vi "Umgebung.ReadZustandsgrössen.vi"(0 "Umgebung in":refnum<data-value>, 5 "error in":errorcluster) -> (14 "Umgebung out":refnum<data-value>, 15 "Sekunden":dbl, 16 "Strahlungsleistung [W]":dbl, 17 "Solare Gewinne [W]":dbl, 18 "Aussentemperatur [°C]":dbl, 19 "error out":errorcluster)   [LabVIEW 2016, in "Umgebung.lvclass"]
uses:
  Umgebung.lvclass
  Umgebung.lvclass/Umgebung.ctl
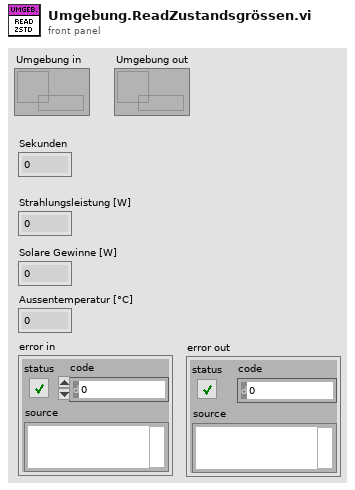
[diagram p1: front panel]
types:
  T1 = typedef "Umgebung.lvclass/Umgebung.Zustandsgrössen.ctl" = cluster{"Aussentemperatur [°C]":dbl, "Aussentemperatur [°C] Manuell":dbl, "Tag":dbl, "Stunde":dbl, "Minute":dbl, "Sekunden":dbl, "Strahlungsleistung [W/m2]":dbl, "Solare Gewinne [W/m2]":dbl, "Solare Gewinne [W/m2] Manuell":dbl, "Manuelle Eingabe On/Off":bool}
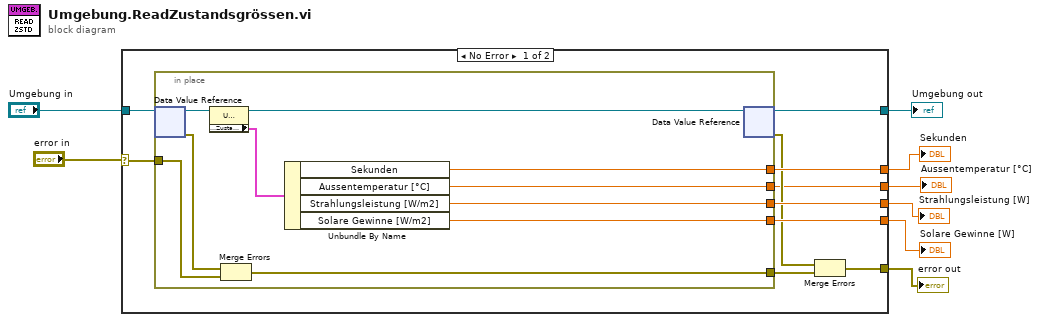
[diagram p0: block diagram]
diagram:
  n1 = case shown="No Error" "error in" {
    selector: "error in" -> [w11 w30]
    tunnel: [w18 _] -> w8
    tunnel: [w17 _] -> w7
    tunnel: "Umgebung in" -> [w16 w29]
    tunnel: [w15 w29] -> w5
    tunnel: [w14 _] -> w4
    tunnel: [w13 w30] -> w2
    tunnel: [w9 _] -> w1
    frame No Error {
      n2 = in-place {
        in-place-border: [w25] -> w18
        in-place-border: [w24] -> w17
        in-place-border: [w23] -> w14
        in-place-border: w11 -> [w21]
        in-place-border: [w20] -> w10
        in-place-border: [w19] -> w9
        n3 = in-place-dvr #1(w16) -> (w28:refnum<class "Umgebung.lvclass">, w22:errorcluster)
        n4 = property class="Umgebung.lvclass"(reference=w28) -> (reference out=w26:refnum<class "Umgebung.lvclass">, "Accessors:Umgebung.Zustandsgrössen"=w27:T1)  [unwired: 1 in, 1 out]
        n5 = Merge Errors(w22, w21) -> (w20:errorcluster)
        n6 = Unbundle By Name(w27) -> ("Sekunden"=w25:dbl, "Aussentemperatur [°C]"=w19:dbl, "Strahlungsleistung [W/m2]"=w24:dbl, "Solare Gewinne [W/m2]"=w23:dbl)
        n7 = in-place-dvr #1(w26) -> (w15:refnum<data-value>, w12:errorcluster)
      }
      n8 = Merge Errors(w12, w10) -> (w13:errorcluster)
    }
    frame Error {
    }
  }
  "Strahlungsleistung [W]" <- w7
  "Sekunden" <- w8
  "Solare Gewinne [W]" <- w4
  "Umgebung out" <- w5
  "error out" <- w2
  "Aussentemperatur [°C]" <- w1
